vi "Populate Categories.vi"(8 "error in (no error)":errorcluster, 10 "Categories":string[](array[string]), 11 "Grid Screen in":refnum<class "Grid Screen.lvclass">) -> (0 "error out":errorcluster, 3 "Grid Screen out":refnum<class "Grid Screen.lvclass">)   [LabVIEW 2024, in "Grid Screen.lvlib" / "Grid Screen.lvclass"]
uses:
  Grid Screen.lvclass
  C:/Program Files/National Instruments/LabVIEW 2024/vi.lib/ActorFramework/Actor/Actor.lvclass
  <vilib>/ActorFramework/Actor/Actor.lvclass/Actor.ctl
  <vilib>/ActorFramework/Message Enqueuer/Message Enqueuer.lvclass/Message Enqueuer.ctl
  Grid Screen.lvclass/Grid Screen.ctl
  Grid Screen Messages/Reset Board Appearance Msg/Reset Board Appearance Msg.lvclass/Reset Board Appearance Msg.ctl
  <vilib>/ActorFramework/Message Enqueuer/Init from Existing Queue.vi
  <vilib>/ActorFramework/Message Enqueuer/Enqueue.vi
  Grid Screen Messages/Reset Board Appearance Msg/Reset Board Appearance Msg.lvclass
  C:/Program Files/National Instruments/LabVIEW 2024/vi.lib/ActorFramework/Message/Message.lvclass
  <vilib>/ActorFramework/Message Priority Queue/Priority Enqueue.vi
  <vilib>/ActorFramework/Message Enqueuer/Message Enqueuer.lvclass
  <vilib>/ActorFramework/Actor/Actor.lvclass
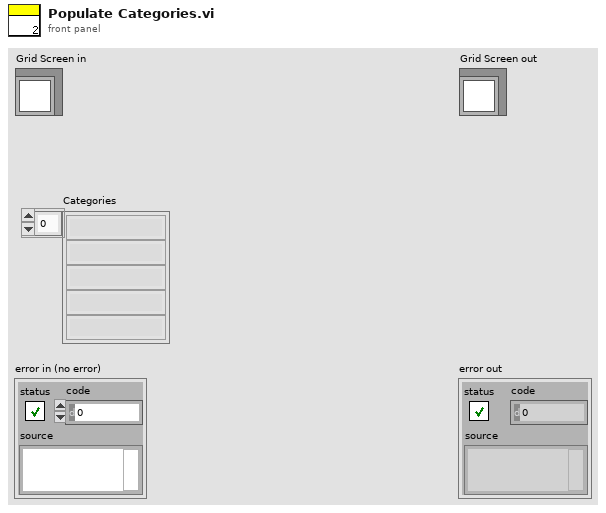
[diagram p1: front panel]
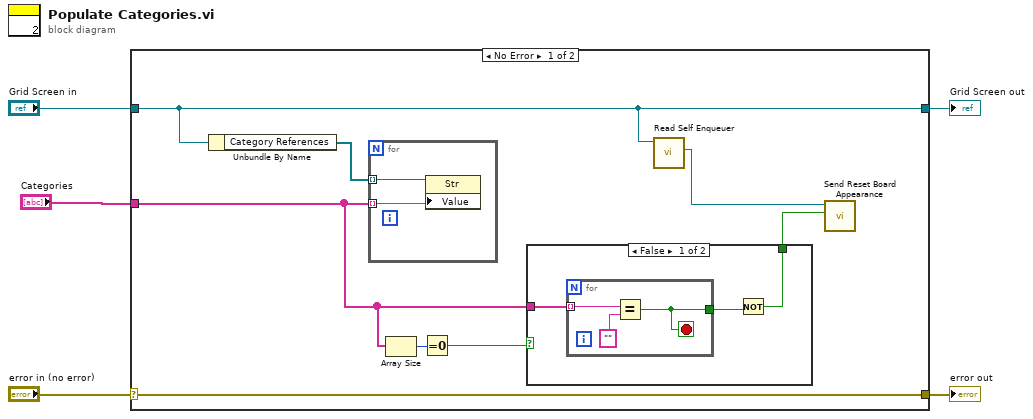
[diagram p0: block diagram]
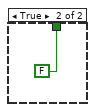
[diagram p2: hidden frame]
diagram:
  n1 = case shown="No Error" "error in (no error)" {
    selector: "error in (no error)" -> [w13 w24]
    tunnel: [w13 w24] -> w4
    tunnel: [w11 w23] -> w2
    tunnel: "Grid Screen in" -> [w11 w23]
    tunnel: "Categories" -> [w6 _]
    frame No Error {
      n2 = Unbundle By Name(w11) -> ("Category References"=w12:refnum<vi>[])
      n3 = for {
        tunnel: w12 -> [w22] mode=indexing
        tunnel: w6 -> [w21] mode=indexing
        n4 = property class="Str"(reference=w22, "Value"=w21) -> ()  [unwired: 1 in, 2 out]
      }
      n5 = Array Size(array=w6) -> (size(s)=w9:i32)
      n6 = Equal To 0?(x=w9) -> (x = 0?=w8:bool)
      n7 = case shown="False" w8 {
        tunnel: [w14 FALSE ("Value")] -> w7
        tunnel: w6 -> [w15 _]
        frame False {
          n8 = for {
            tunnel: w15 -> [w19] mode=indexing
            tunnel: [w17] -> w16
            stop <- w17 stop-if-true
            n9 = Equal?(x=w19, y="") -> (x = y?=w17:bool)
          }
          n10 = Not(x=w16) -> (.not. x?=w14:bool)
        }
        frame True {
        }
      }
      n11 = call <vilib>:"Read Self Enqueuer.vi"("Actor"=w11) -> ("Self Enqueuer"=w10:refnum<class "Message Enqueuer.lvclass">)  [unwired: 10 in]
      n12 = call "Send Reset Board Appearance.vi"("Value"=w7, "Message Enqueuer"=w10) -> ()  [unwired: 8 in, 2 out]
    }
    frame Error {
    }
  }
  "error out" <- w4
  "Grid Screen out" <- w2
